vi "Acquire.vi"(8 "error in (no error)":errorcluster, 10 "Units":i32(ring) items=["degC", "degF", "kelvin", "raw"], 11 "physical channels":refnum<k21>) -> (0 "error out":errorcluster, 2 "Graph Data":waveform(dbl)[](array[waveform]))   [LabVIEW 2020, in "GetTemperature.lvlib"]
doc: "Perform the acquisition. Replace the contents of this diagram with calls to acquisition hardware.\n_____\nBased on Delacor QMH Project Template 5.0.0.82."
uses:
  GetTemperature.lvlib
  <vilib>/ULx/Create Channel.llb/ULx Create Channel (AI-Temperature).vi
  <vilib>/ULx/Read.llb/ULx Read (Analog Wfm 1Chan 1Samp).vi
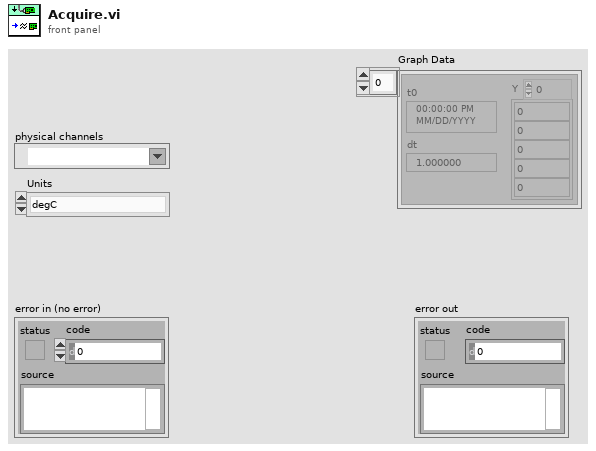
[diagram p1: front panel]
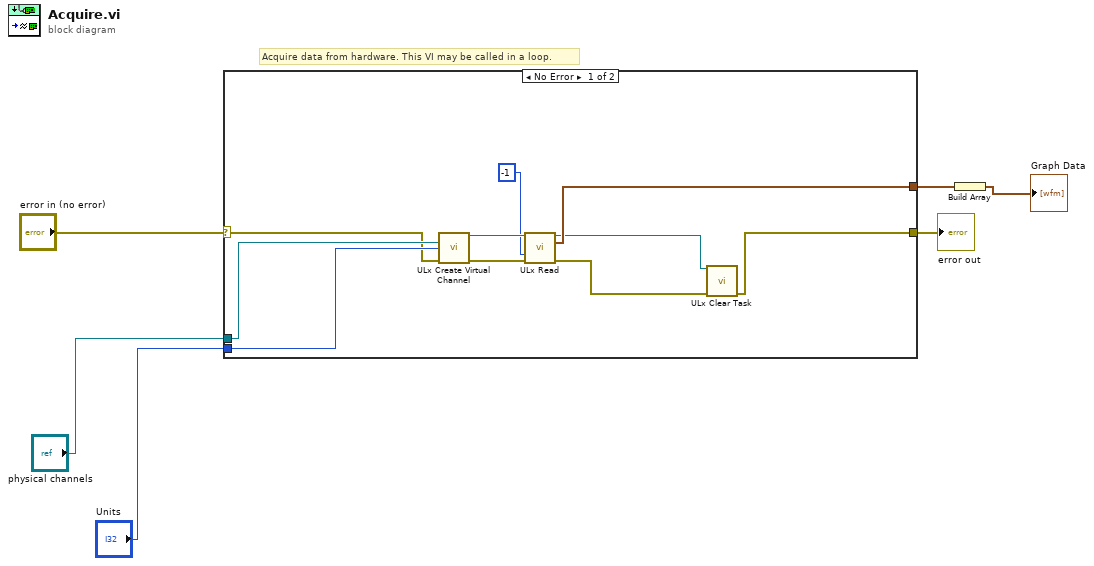
[diagram p0: block diagram]
diagram:
  # "Acquire data from hardware. This VI may be called in a loop."
  n1 = case shown="No Error" "error in (no error)" {
    selector: "error in (no error)" -> [w14 w17]
    tunnel: [w8 w17] -> w5
    tunnel: "Units" -> [w15 _]
    tunnel: "physical channels" -> [w16 _]
    tunnel: [w11 _] -> w2
    frame No Error {
      n2 = call-poly <vilib>:"ULx Create Virtual Channel.vi"("physical channels"=w16, "units"=w15, "error in"=w14) -> ("task out"=w13:refnum<k24>, "error out"=w12:errorcluster)  [unwired: 11 in]
      n3 = call-poly <vilib>:"ULx Read.vi"("task in"=w13, "timeout"=-1, "error in"=w12) -> ("task out"=w10:refnum<k24>, "data"=w11:waveform(dbl), "error out"=w9:errorcluster)  [unwired: 10 in]
      n4 = call <vilib>:"ULx Clear Task.vi"("task in"=w10, "error in"=w9) -> ("error out"=w8:errorcluster)  [unwired: 13 in]
    }
    frame Error {
    }
  }
  "error out" <- w5
  n5 = Build Array(w2) -> (→"Graph Data":waveform(dbl)[])
